vi "Constants.vi"() -> ()   [LabVIEW 2015, in "TestStand Analysis Steps.lvlib"]
uses:
  TestStand Analysis Steps.lvlib
panel:
  in  "Result.Prefix":string="Result." caption="Result.Prefix (DO NOT CHANGE)"
  in  "SN.Sufix":string=".SerialNumber"
  in  "VBATT.Property":string="VBATT"
  in  "Cycled.Sufix":string=".Cycled"
  in  "LT.AnalyzeChannel":string="LT.AnalyzeChannel"
  in  "Rate.Property":string="LogRate"
  in  "LT.Sufix":string="LevelTransition"
  in  "VS Group":string="VeriStand Channels"
  in  "Iteration.Property":string="Iteration" caption="Iteration.Property (DO NOT CHANGE)"
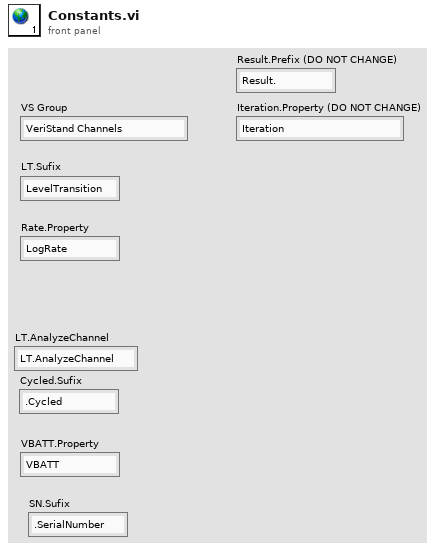
[diagram p1: front panel]
diagram:
